vi "RecordingStart.vi"(11 "Connection ID":T1) -> (3 "Connection ID Out":T1)   [LabVIEW 2017, in "GL860_Driver.lvlib"]
uses:
  GL860_Driver.lvlib
  Driver/ConnectionID.ctl
panel:
  in  "閉じる":bool
  in  "収録ファイルパス":path
  in  "OneShot":bool
  in  "Stop":bool
  in  "Start":bool
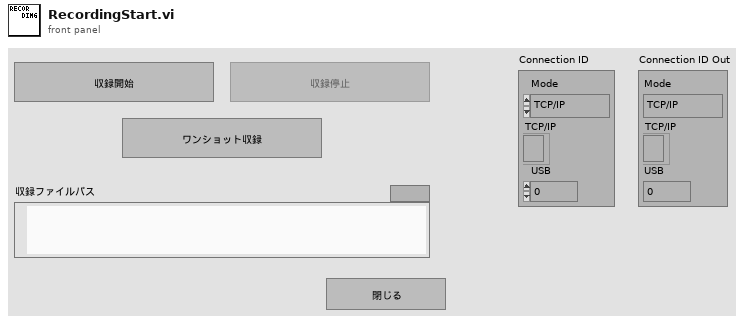
[diagram p1: front panel]
types:
  T1 = typedef "ConnectionID.ctl" = cluster{"Mode":enum16{"TCP/IP", "USB"}, "TCP/IP":refnum<k5>, "USB":i32}
  T2 = enum16{"open", "replace", "create", "open or create", "replace or create", "replace or create with confirmation"}
  T3 = typedef "Amp_Param.ctl" = cluster{"File":refnum<file>[], "Idx":refnum<file>[], "dT":dbl, "Hd":i32, "Rd":i32, "Start":timestamp[], "Trig":timestamp[], "Stop":timestamp[], "FirstPos":timestamp[], "Count":i64[], "Color":u32[], "Label":string[], "INP":string[], "H":dbl[], "L":dbl[], "Fmt":string[], "Unit":string[], "SEL":i32[], "Byte":i32[], "Pos":i32[], "Bit":i32[], "Flg":i32[], "Gain":dbl[], "Offset":dbl[], "CH":i32[], "Opt":cluster{"Mode":i32, "TUNIT":enum16{"CELS", "FAHR"}}, "TYPE":enum16{"GBD", "CSV"}, "Comp":refnum<file>[], "Temp":i32[]}
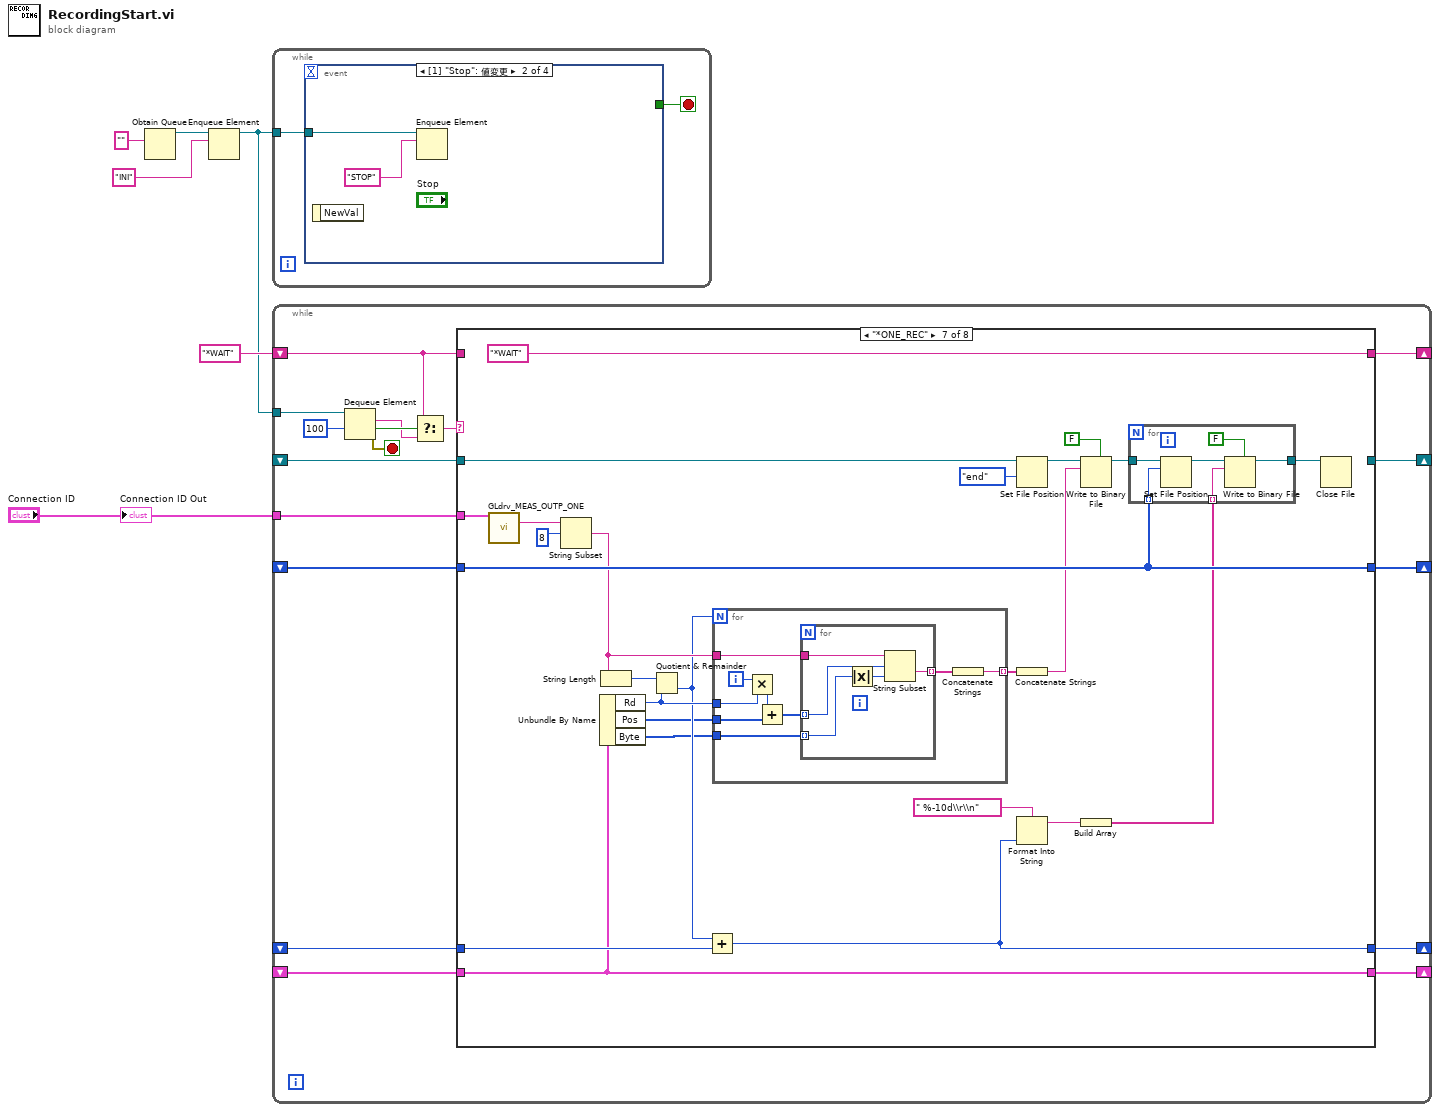
[diagram p0: block diagram]
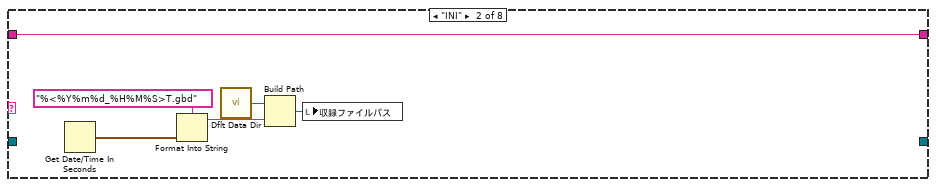
[diagram p3: hidden frame]
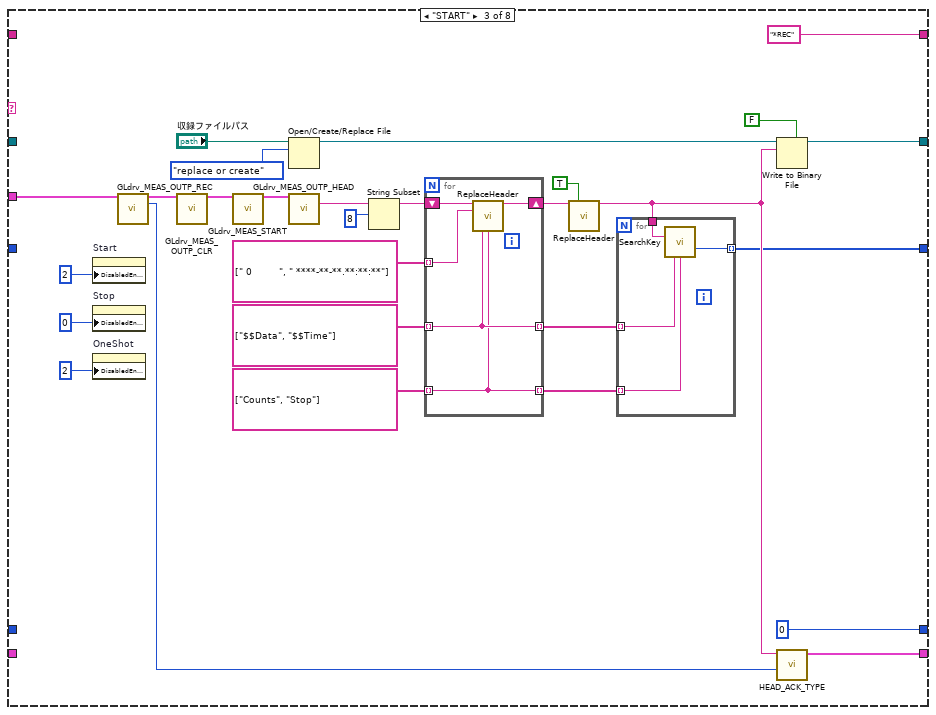
[diagram p4: hidden frame]
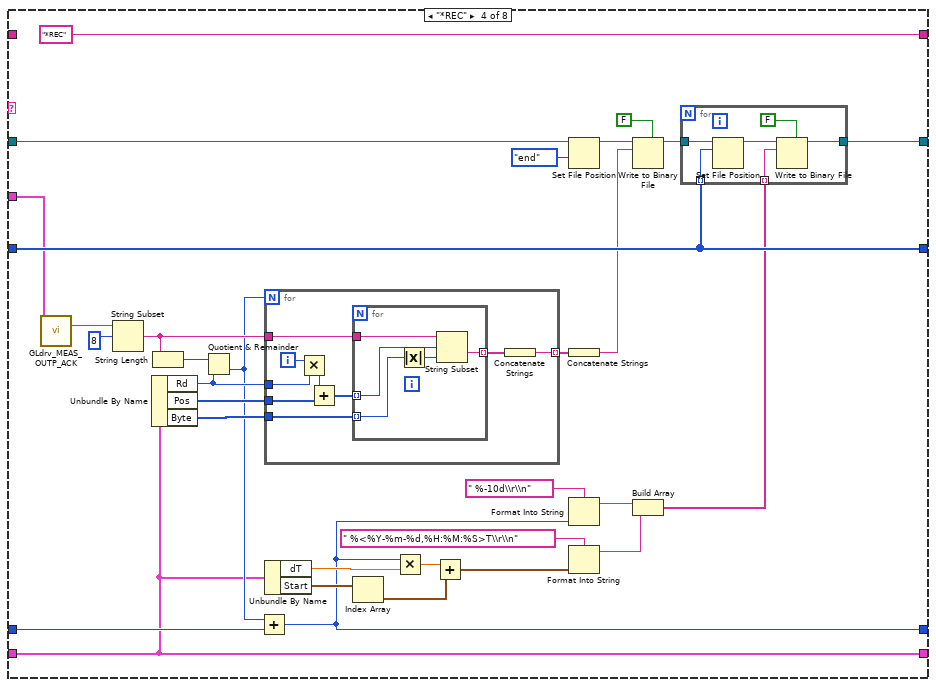
[diagram p5: hidden frame]
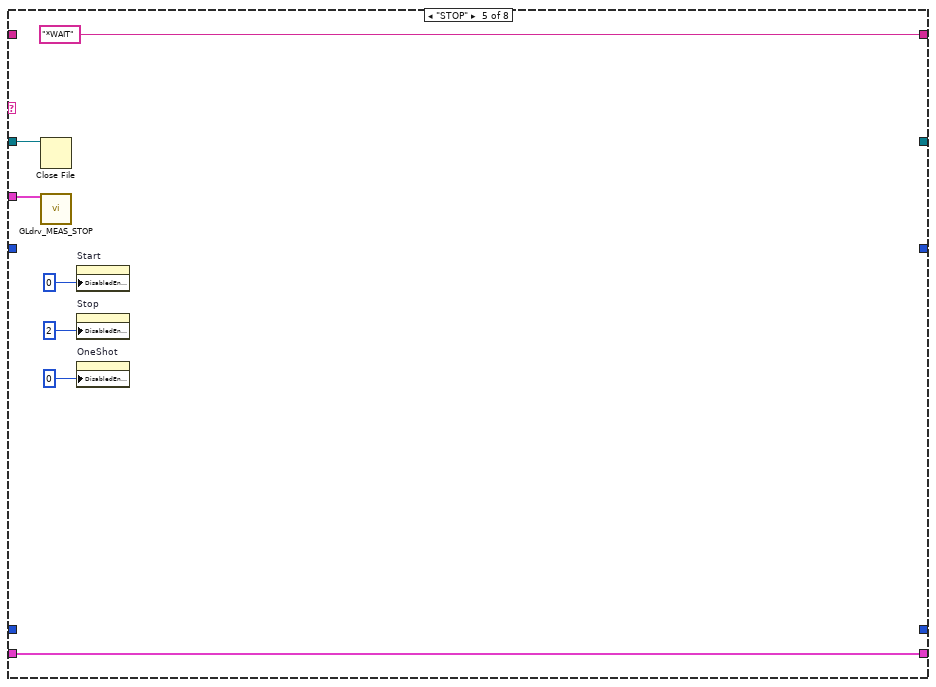
[diagram p6: hidden frame]
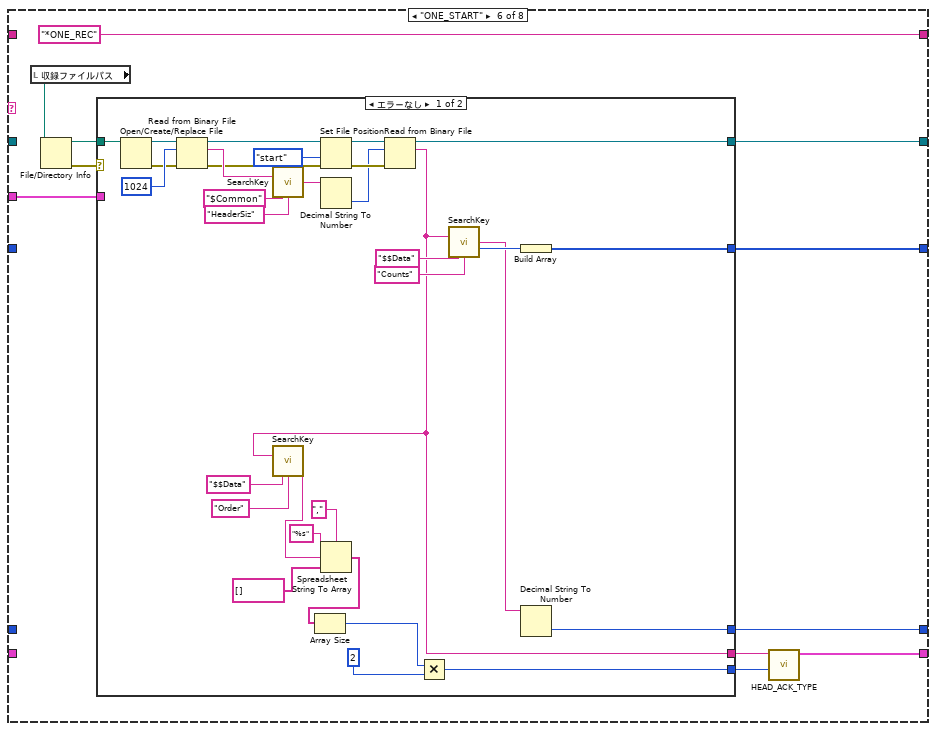
[diagram p7: hidden frame]
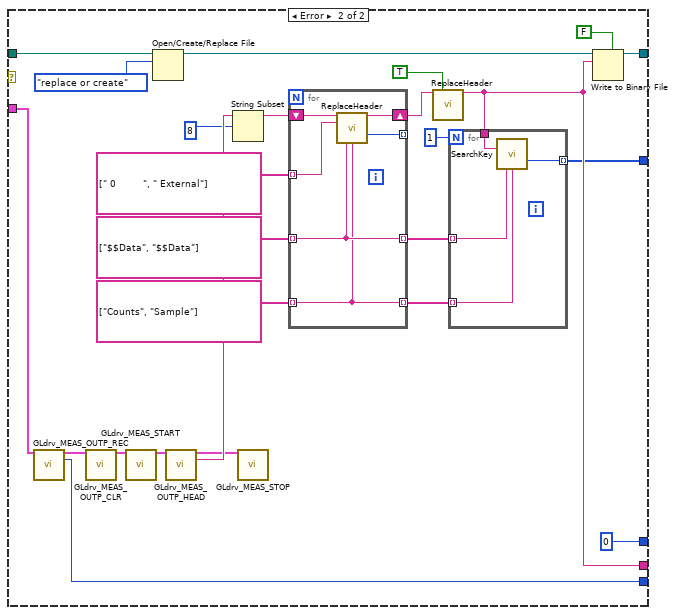
[diagram p8: hidden frame]
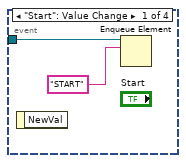
[diagram p10: hidden frame]
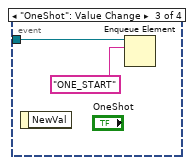
[diagram p11: hidden frame]
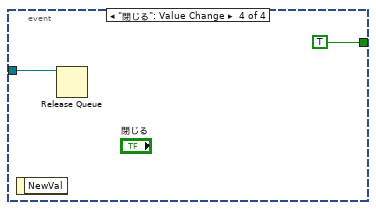
[diagram p12: hidden frame]
diagram:
  n1 = Obtain Queue(element data type="") -> (queue out=w2:refnum<queue>)  [unwired: 4 in, 2 out]
  n2 = Enqueue Element(queue=w2, element="INI") -> (queue out=w3:refnum<queue>)  [unwired: 2 in, 2 out]
  n3 = while {
    tunnel: w3 -> [w7]
    stop <- w8 stop-if-true
    n4 = event shown="[1] \"Stop\": 値変更" {
      selector: _ -> [_ _ _ _]
      dyn-events: _ -> [_ _ _ _]
      timeout: _ -> [_ _ _ _]
      tunnel: [_ _ _ TRUE] -> w8
      tunnel: w7 -> [w9 w11 w13 w15]
      event "Start": Value Change {
        n5 = event-data() -> ()  [unwired: 1 in, 1 out]
        n6 = Enqueue Element(queue=w9, element="START") -> ()  [unwired: 2 in, 3 out]
      }
      event "Stop": Value Change {
        n7 = event-data() -> ()  [unwired: 1 in, 1 out]
        n8 = Enqueue Element(queue=w11, element="STOP") -> ()  [unwired: 2 in, 3 out]
      }
      event "OneShot": Value Change {
        n9 = event-data() -> ()  [unwired: 1 in, 1 out]
        n10 = Enqueue Element(queue=w13, element="ONE_START") -> ()  [unwired: 2 in, 3 out]
      }
      event "閉じる": Value Change {
        n11 = event-data() -> ()  [unwired: 1 in, 1 out]
        n12 = Release Queue(queue=w15) -> ()  [unwired: 2 in, 3 out]
      }
    }
  }
  n13 = while {
    tunnel: "Connection ID" -> [w33]
    tunnel: w3 -> [w30]
    shift-right: [w27] -> _
    shift-left: "*WAIT" -> [w24]
    shift-right: [w28] -> _
    shift-left: _ -> [w26]
    shift-right: [w22] -> _
    shift-left: _ -> [w21]
    shift-right: [w19] -> _
    shift-left: _ -> [w20]
    shift-right: [w18] -> _
    shift-left: _ -> [w17]
    stop <- w23 stop-if-true
    n14 = Dequeue Element(queue=w30, timeout in ms (-1)=100) -> (element=w31:string, timed out?=w32:bool, error out=w23:errorcluster)  [unwired: 1 in, 1 out]
    n15 = Select(t=w24, s=w32, f=w31) -> (s? t:f=w29:string)
    n16 = case shown="\"*ONE_REC\"" w29 {
      tunnel: w33 -> [_ _ w47 w85 w135 w151 w234 _]
      tunnel: [w37 _ w70 w86 _ w150 _ _] -> w28
      tunnel: [w38 w40 "*REC" "*REC" "*WAIT" "*ONE_REC" "*WAIT" _] -> w27
      tunnel: w26 -> [w37 _ _ w99 w140 _ w223 _]
      tunnel: w24 -> [w38 w40 _ _ _ _ _ _]
      tunnel: [w36 _ w49 w113 _ w149 w243 _] -> w22
      tunnel: w21 -> [w36 _ _ w113 _ _ w243 _]
      tunnel: w20 -> [w34 _ _ w109 _ _ w237 _]
      tunnel: [w34 _ 0 w89 _ w147 w235 _] -> w19
      tunnel: [w35 _ w55 w87 w134 w143 w226 _] -> w18
      tunnel: w17 -> [w35 _ _ w87 w134 _ w226 _]
      frame Default {
      }
      frame "INI" {
        n17 = Get Date/Time In Seconds() -> (seconds since 1Jan1904=w42:timestamp)
        n18 = Format Into String(format string="%<%Y%m%d_%H%M%S>T.gbd" ("name or relative path"), w42) -> (resulting string=w43:string)  [unwired: 2 in, 1 out]
        n19 = call <vilib>:"Dflt Data Dir.vi"() -> ("App:Default Data Directory"=w39:path)
        n20 = Build Path(base path=w39, name or relative path=w43) -> (appended path=w41:path)
        n21 = local write "収録ファイルパス"(w41) -> ()
      }
      frame "START" {
        n22 = property on="Start" class="Bool"("DisabledEnum"=u16 2) -> ()  [unwired: 2 in, 2 out]
        n23 = property on="Stop" class="Bool"("DisabledEnum"=u16 0) -> ()  [unwired: 2 in, 2 out]
        n24 = property on="OneShot" class="Bool"("DisabledEnum"=u16 2) -> ()  [unwired: 2 in, 2 out]
        n25 = call "GLdrv_MEAS_OUTP_REC.vi"("Connection ID"=w47) -> ("Connection ID Out"=w46:T1, "ACK Size out"=w45:i32)  [unwired: 12 in, 1 out]
        n26 = call "GLdrv_MEAS_OUTP_CLR.vi"("Connection ID"=w46) -> ("Connection ID Out"=w71:T1)  [unwired: 12 in, 2 out]
        n27 = call "GLdrv_MEAS_START.vi"("Connection ID"=w71) -> ("Connection ID Out"=w72:T1)  [unwired: 13 in, 1 out]
        n28 = Open/Create/Replace File(file path (use dialog)="収録ファイルパス", operation (0:open)=T2."replace or create") -> (refnum out=w61:refnum<file>)  [unwired: 4 in, 2 out]
        n29 = call "GLdrv_MEAS_OUTP_HEAD.vi"("Connection ID"=w72) -> ("Header out"=w65:string)  [unwired: 12 in, 2 out]
        n30 = String Subset(string=w65, offset (0)=8) -> (substring=w48:string)  [unwired: 1 in]
        n31 = for {
          tunnel: string[] ["$$Data", "$$Time"] -> [w78] mode=indexing
          tunnel: string[] ["Counts", "Stop"] -> [w77] mode=indexing
          tunnel: string[] [" 0         ", " ****-**-**.**:**:**"] -> [w79] mode=indexing
          shift-right: [w80] -> w54
          shift-left: w48 -> [w81]
          tunnel: [w78] -> w51 mode=indexing
          tunnel: [w77] -> w50 mode=indexing
          n32 = call "ReplaceHeader.vi"("In"=w81, "string"=w79, "KEY1"=w78, "KEY2"=w77) -> ("Out"=w80:string)  [unwired: 9 in, 2 out]
        }
        n33 = call "ReplaceHeader.vi"("In"=w54, "Size"=TRUE) -> ("Out"=w52:string)  [unwired: 11 in, 2 out]
        n34 = for {
          tunnel: w52 -> [w76]
          tunnel: w51 -> [w75] mode=indexing
          tunnel: w50 -> [w74] mode=indexing
          tunnel: [w73] -> w49 mode=indexing
          n35 = call "SearchKey.vi"("In"=w76, "KEY1"=w75, "KEY2"=w74) -> ("Position"=w73:i32)  [unwired: 12 out]
        }
        n36 = Write to Binary File(file (use dialog)=w61, data=w52, 5:FALSE ("prepend array or string size? (T)")) -> (refnum out=w70:refnum<file>)  [unwired: 3 in, 2 out]
        n37 = call "HEAD_ACK_TYPE.vi"("Record"=w45, "GBD"=w52) -> ("output cluster"=w55:T3)  [unwired: 9 in]
      }
      frame "*REC" {
        n38 = call "GLdrv_MEAS_OUTP_ACK.vi"("Connection ID"=w85) -> ("Data out"=w84:string)  [unwired: 12 in, 2 out]
        n39 = String Subset(string=w84, offset (0)=8) -> (substring=w102:string)  [unwired: 1 in]
        n40 = Unbundle By Name(w87) -> ("Rd"=w106:i32, "Pos"=w103:i32[], "Byte"=w104:i32[])
        n41 = String Length(string=w102) -> (length=w105:i32)
        n42 = Quotient & Remainder(x=w105, y=w106) -> (floor(x/y)=w101:i32)  [unwired: 1 out]
        n43 = Add(x=w101, y=w109) -> (x+y=w89:i32)
        n44 = for {
          N: w101 -> [_]
          tunnel: w102 -> [w122]
          tunnel: w103 -> [w117]
          tunnel: w104 -> [w121]
          tunnel: w106 -> [w120]
          tunnel: [w114] -> w82 mode=indexing
          i -> [w119]
          n45 = Multiply(x=w119, y=w120) -> (x*y=w118:i32)
          n46 = Add(x=w118, y=w117) -> (x+y=w116:i32[])
          n47 = for {
            tunnel: w121 -> [w126] mode=indexing
            tunnel: w122 -> [w127]
            tunnel: w116 -> [w124] mode=indexing
            tunnel: [w123] -> w115 mode=indexing
            n48 = Absolute Value(x=w126) -> (abs(x)=w125:i32)
            n49 = String Subset(string=w127, offset (0)=w124, length (rest)=w125) -> (substring=w123:string)
          }
          n50 = Concatenate Strings(w115) -> (w114:string)
        }
        n51 = Unbundle By Name(w87) -> ("dT"=w92:dbl, "Start"=w91:timestamp[])
        n52 = Index Array(array=w91) -> (element=w90:timestamp)  [unwired: 1 in]
        n53 = Multiply(x=w89, y=w92) -> (x*y=w93:dbl)
        n54 = Add(x=w93, y=w90) -> (x+y=w94:timestamp)
        n55 = Set File Position(refnum=w99, from (0:start)=enum16{"start", "end", "current"}."end") -> (refnum out=w112:refnum<file>)  [unwired: 2 in, 1 out]
        n56 = Concatenate Strings(w82) -> (w83:string)
        n57 = Format Into String(format string=" %-10d\\r\\n", w89) -> (resulting string=w96:string)  [unwired: 2 in, 1 out]
        n58 = Format Into String(format string=" %<%Y-%m-%d,%H:%M:%S>T\\r\\n", w94) -> (resulting string=w95:string)  [unwired: 2 in, 1 out]
        n59 = Write to Binary File(file (use dialog)=w112, data=w83, 5:FALSE ("prepend array or string size? (T)")) -> (refnum out=w100:refnum<file>)  [unwired: 3 in, 2 out]
        n60 = Build Array(w96, w95) -> (w88:string[])
        n61 = for {
          tunnel: w100 -> [w132]
          tunnel: [w133] -> w86
          tunnel: w113 -> [w130] mode=indexing
          tunnel: w88 -> [w129] mode=indexing
          n62 = Set File Position(offset (in bytes) (0)=w130, refnum=w132) -> (refnum out=w131:refnum<file>)  [unwired: 2 in, 1 out]
          n63 = Write to Binary File(file (use dialog)=w131, data=w129, 5:FALSE ("prepend array or string size? (T)")) -> (refnum out=w133:refnum<file>)  [unwired: 3 in, 2 out]
        }
      }
      frame "STOP" {
        n64 = Close File(refnum=w140) -> ()  [unwired: 1 in, 2 out]
        n65 = call "GLdrv_MEAS_STOP.vi"("Connection ID"=w135) -> ()  [unwired: 13 in, 2 out]
        n66 = property on="Start" class="Bool"("DisabledEnum"=u16 0) -> ()  [unwired: 2 in, 2 out]
        n67 = property on="Stop" class="Bool"("DisabledEnum"=u16 2) -> ()  [unwired: 2 in, 2 out]
        n68 = property on="OneShot" class="Bool"("DisabledEnum"=u16 0) -> ()  [unwired: 2 in, 2 out]
      }
      frame "ONE_START" {
        n69 = local read "収録ファイルパス"() -> (w146:path)
        n70 = File/Directory Info(path=w146) -> (path out=w144:path, error out=w145:errorcluster)  [unwired: 1 in, 5 out]
        n71 = case shown="エラーなし" w145 {
          tunnel: w151 -> [_ w186]
          tunnel: [w169 w208] -> w150
          tunnel: [w166 w191] -> w149
          tunnel: [w163 0] -> w147
          tunnel: [w153 w195] -> w142
          tunnel: w144 -> [w170 w198]
          tunnel: [w152 w184] -> w141
          frame No Error {
            n72 = Open/Create/Replace File(file path (use dialog)=w170) -> (refnum out=w175:refnum<file>, error out=w174:errorcluster)  [unwired: 1 in, 5 out]
            n73 = Read from Binary File(8:w174, 10:1024 ("count"), 11:w175) -> (0:w171:errorcluster, 2:w172:string, 3:w181:refnum<file>)  [unwired: 4 out]
            n74 = call "SearchKey.vi"("In"=w172, "KEY1"="$Common", "KEY2"="HeaderSiz") -> ("String"=w178:string)  [unwired: 12 out]
            n75 = Set File Position(refnum=w181, from (0:start)=enum16{"start", "end", "current"}."start" ("pos mode (0:2)"), error in=w171) -> (refnum out=w177:refnum<file>, error out=w176:errorcluster)  [unwired: 1 out]
            n76 = Decimal String To Number(string=w178) -> (number=w173:i32)  [unwired: 3 out]
            n77 = Read from Binary File(8:w176, 10:w173, 11:w177) -> (2:w153:string, 3:w169:refnum<file>)  [unwired: 5 out]
            n78 = call "SearchKey.vi"("In"=w153, "KEY1"="$$Data", "KEY2"="Order") -> ("String"=w158:string)  [unwired: 12 out]
            n79 = Spreadsheet String To Array(delimiter (Tab)=",", format string="%s", spreadsheet string=w158, array type (2D Dbl)=string[] []) -> (array=w157:string[])
            n80 = Array Size(array=w157) -> (size(s)=w156:i32)
            n81 = Multiply(x=w156, y=2) -> (x*y=w152:i32)
            n82 = call "SearchKey.vi"("In"=w153, "KEY1"="$$Data", "KEY2"="Counts") -> ("String"=w164:string, "Position"=w165:i32)  [unwired: 11 out]
            n83 = Build Array(w165) -> (w166:i32[])
            n84 = Decimal String To Number(string=w164) -> (number=w163:i32)  [unwired: 2 in, 1 out]
          }
          frame Error {
            n85 = call "GLdrv_MEAS_OUTP_REC.vi"("Connection ID"=w186) -> ("Connection ID Out"=w185:T1, "ACK Size out"=w184:i32)  [unwired: 12 in, 1 out]
            n86 = call "GLdrv_MEAS_OUTP_CLR.vi"("Connection ID"=w185) -> ("Connection ID Out"=w188:T1)  [unwired: 12 in, 2 out]
            n87 = call "GLdrv_MEAS_START.vi"("Connection ID"=w188) -> ("Connection ID Out"=w189:T1)  [unwired: 13 in, 1 out]
            n88 = Open/Create/Replace File(file path (use dialog)=w198, operation (0:open)=T2."replace or create") -> (refnum out=w199:refnum<file>)  [unwired: 4 in, 2 out]
            n89 = call "GLdrv_MEAS_OUTP_HEAD.vi"("Connection ID"=w189) -> ("Connection ID Out"=w187:T1, "Header out"=w202:string)  [unwired: 12 in, 1 out]
            n90 = String Subset(string=w202, offset (0)=8) -> (substring=w190:string)  [unwired: 1 in]
            n91 = call "GLdrv_MEAS_STOP.vi"("Connection ID"=w187) -> ()  [unwired: 13 in, 2 out]
            n92 = for {
              tunnel: string[] ["$$Data", "$$Data"] -> [w214] mode=indexing
              tunnel: string[] ["Counts", "Sample"] -> [w213] mode=indexing
              tunnel: string[] [" 0         ", " External"] -> [w215] mode=indexing
              shift-right: [w216] -> w197
              shift-left: w190 -> [w217]
              tunnel: [w218] -> _ mode=indexing
              tunnel: [w214] -> w194 mode=indexing
              tunnel: [w213] -> w193 mode=indexing
              n93 = call "ReplaceHeader.vi"("In"=w217, "string"=w215, "KEY1"=w214, "KEY2"=w213) -> ("Out"=w216:string, "StartPos"=w218:i32)  [unwired: 9 in, 1 out]
            }
            n94 = call "ReplaceHeader.vi"("In"=w197, "Size"=TRUE) -> ("Out"=w195:string)  [unwired: 11 in, 2 out]
            n95 = for {
              N: 1 -> [_]
              tunnel: w195 -> [w212]
              tunnel: w194 -> [w211] mode=indexing
              tunnel: w193 -> [w210] mode=indexing
              tunnel: [w209] -> w191 mode=indexing
              n96 = call "SearchKey.vi"("In"=w212, "KEY1"=w211, "KEY2"=w210) -> ("Position"=w209:i32)  [unwired: 12 out]
            }
            n97 = Write to Binary File(file (use dialog)=w199, data=w195, 5:FALSE ("prepend array or string size? (T)")) -> (refnum out=w208:refnum<file>)  [unwired: 3 in, 2 out]
          }
        }
        n98 = call "HEAD_ACK_TYPE.vi"("Record"=w141, "GBD"=w142) -> ("output cluster"=w143:T3)  [unwired: 9 in]
      }
      frame "*ONE_REC" {
        n99 = call "GLdrv_MEAS_OUTP_ONE.vi"("Connection ID"=w234) -> ("Data out"=w233:string)  [unwired: 12 in, 2 out]
        n100 = String Subset(string=w233, offset (0)=8) -> (substring=w228:string)  [unwired: 1 in]
        n101 = Unbundle By Name(w226) -> ("Rd"=w231:i32, "Pos"=w221:i32[], "Byte"=w220:i32[])
        n102 = String Length(string=w228) -> (length=w230:i32)
        n103 = Quotient & Remainder(x=w230, y=w231) -> (floor(x/y)=w227:i32)  [unwired: 1 out]
        n104 = Add(x=w227, y=w237) -> (x+y=w235:i32)
        n105 = for {
          N: w227 -> [_]
          tunnel: w228 -> [w252]
          tunnel: w221 -> [w247]
          tunnel: w220 -> [w251]
          tunnel: w231 -> [w250]
          tunnel: [w244] -> w222 mode=indexing
          i -> [w249]
          n106 = Multiply(x=w249, y=w250) -> (x*y=w248:i32)
          n107 = Add(x=w248, y=w247) -> (x+y=w246:i32[])
          n108 = for {
            tunnel: w251 -> [w256] mode=indexing
            tunnel: w252 -> [w257]
            tunnel: w246 -> [w254] mode=indexing
            tunnel: [w253] -> w245 mode=indexing
            n109 = Absolute Value(x=w256) -> (abs(x)=w255:i32)
            n110 = String Subset(string=w257, offset (0)=w254, length (rest)=w255) -> (substring=w253:string)
          }
          n111 = Concatenate Strings(w245) -> (w244:string)
        }
        n112 = Set File Position(refnum=w223, from (0:start)=enum16{"start", "end", "current"}."end") -> (refnum out=w242:refnum<file>)  [unwired: 2 in, 1 out]
        n113 = Concatenate Strings(w222) -> (w219:string)
        n114 = Format Into String(format string=" %-10d\\r\\n", w235) -> (resulting string=w239:string)  [unwired: 2 in, 1 out]
        n115 = Write to Binary File(file (use dialog)=w242, data=w219, 5:FALSE ("prepend array or string size? (T)")) -> (refnum out=w225:refnum<file>)  [unwired: 3 in, 2 out]
        n116 = Build Array(w239) -> (w229:string[])
        n117 = for {
          tunnel: w225 -> [w262]
          tunnel: [w263] -> w224
          tunnel: w243 -> [w260] mode=indexing
          tunnel: w229 -> [w259] mode=indexing
          n118 = Set File Position(offset (in bytes) (0)=w260, refnum=w262) -> (refnum out=w261:refnum<file>)  [unwired: 2 in, 1 out]
          n119 = Write to Binary File(file (use dialog)=w261, data=w259, 5:FALSE ("prepend array or string size? (T)")) -> (refnum out=w263:refnum<file>)  [unwired: 3 in, 2 out]
        }
        n120 = Close File(refnum=w224) -> ()  [unwired: 1 in, 2 out]
      }
      frame "EXIT" {
      }
    }
  }
  "Connection ID Out" <- "Connection ID"
